vi "Set Optimiser Parameters and Observables.vi"(0 "Optimiser Cell in":refnum<class "Optimiser Cell.lvclass">, 5 "Parameters":T3[](array[typedef]), 7 "Parameters - string":T1[](array[typedef]), 9 "Observables":T2[](array[typedef]) {"Weight" min=0.0 max=1.0}, 11 "error in (no error)":errorcluster, 12 "Number of Exploration Runs":i32) -> (4 "Optimiser Cell out":refnum<class "Optimiser Cell.lvclass">, 15 "error out":errorcluster)   [LabVIEW 2020, in "Run Utilities.lvlib" / "Optimiser Cell.lvclass"]
uses:
  Optimiser Cell.lvclass
  Optimise parameter - numeric.ctl
  Optimisation observable.ctl
  Optimise parameter - string.ctl
  Optimiser Cell.lvclass/Optimiser Cell.ctl
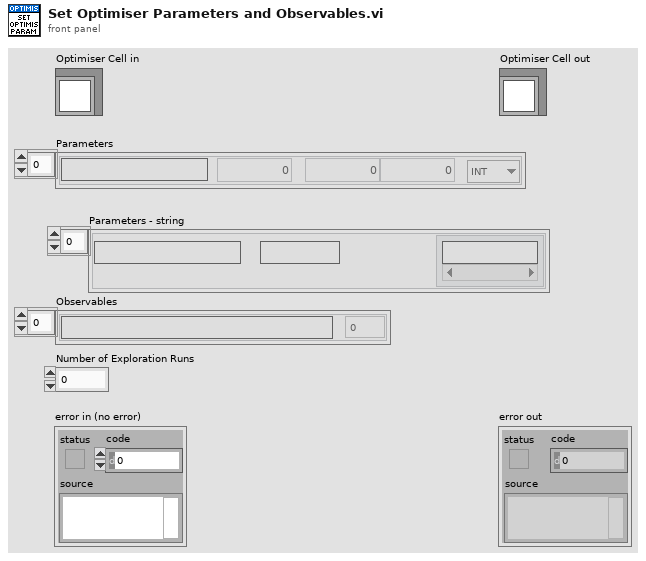
[diagram p1: front panel]
types:
  T1 = typedef "Run Utilities.lvlib/Optimiser Cell.lvclass/Optimise parameter - string.ctl" = cluster{"Name":string, "Start value":string, "Options":string[]}
  T2 = typedef "Run Utilities.lvlib/Optimiser Cell.lvclass/Optimisation observable.ctl" = cluster{"Name":string, "Weight":dbl}
  T3 = typedef "Run Utilities.lvlib/Optimiser Cell.lvclass/Optimise parameter - numeric.ctl" = cluster{"Name":string, "Start value":dbl, "From":dbl, "To":dbl, "dtype":enum16{"INT", "DBL"}}
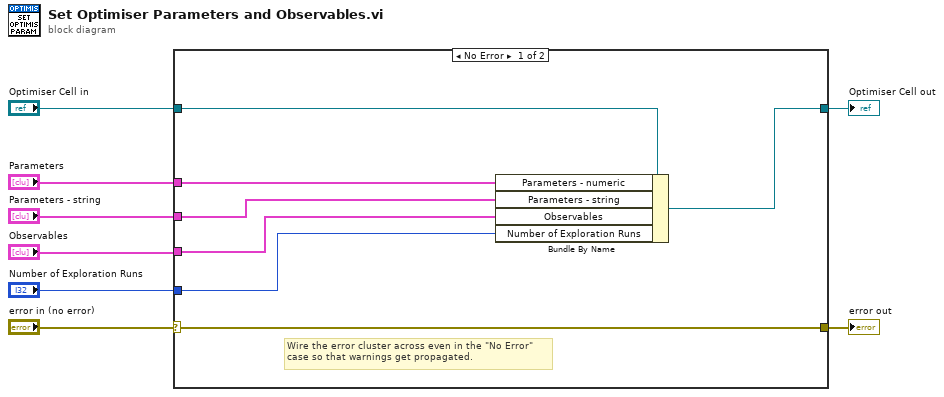
[diagram p0: block diagram]
diagram:
  n1 = case shown="No Error" "error in (no error)" {
    selector: "error in (no error)" -> [w15 w17]
    tunnel: [w15 w17] -> w7
    tunnel: [w13 w16] -> w5
    tunnel: "Optimiser Cell in" -> [w14 w16]
    tunnel: "Parameters" -> [w12 _]
    tunnel: "Observables" -> [w10 _]
    tunnel: "Parameters - string" -> [w11 _]
    tunnel: "Number of Exploration Runs" -> [w9 _]
    frame No Error {
      # "Wire the error cluster across even in the \"No Error\"\ncase so that warnings get propagated."
      n2 = Bundle By Name(cluster=w14, "Parameters - numeric"=w12, "Parameters - string"=w11, "Observables"=w10, "Number of Exploration Runs"=w9) -> (w13:refnum<class "Optimiser Cell.lvclass">)
    }
    frame Error {
    }
  }
  "error out" <- w7
  "Optimiser Cell out" <- w5
